vi "Motor Controler.vi"() -> ()   [LabVIEW 2018]
panel:
  in  "Voltage":dbl(knob) scale=0.0..2.0
  out "Motor":dbl(knob) scale=0.0..9.0
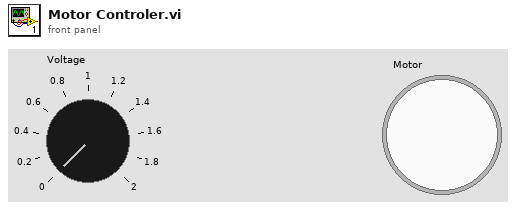
[diagram p1: front panel]
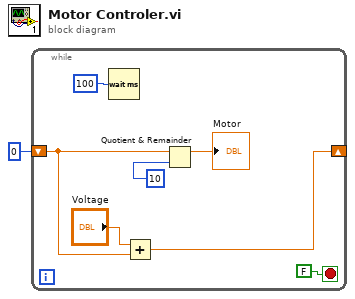
[diagram p0: block diagram]
diagram:
  n1 = while {
    shift-right: [w4] -> _
    shift-left: 0 -> [w5]
    stop <- FALSE stop-if-true
    n2 = Wait (ms)(milliseconds to wait=u32 100) -> ()  [unwired: 1 out]
    n3 = Add(x="Voltage", y=w5) -> (x+y=w4:dbl)
    n4 = Quotient & Remainder(x=w5, y=10) -> (x-y*floor(x/y)=→"Motor":dbl)  [unwired: 1 out]
  }
